vi "DPO_7K_Read Multiple Waveforms.vi"(8 "error in (no error)":errorcluster, 10 "Channels":u16[](array[ring])=[0] items=["Channel 1", "Channel 2", "Channel 3", "Channel 4", "Math 1", "Math 2", "Math 3", "Math 4", "Reference 1", "Reference 2", "Reference 3", "Reference 4"], 11 "VISA resource name":refnum<visa-resource-name>) -> (0 "error out":errorcluster, 1 "ChannelsArray":u16[](array[ring]) caption="Channels" items=["Channel 1", "Channel 2", "Channel 3", "Channel 4", "Math 1", "Math 2", "Math 3", "Math 4", "Reference 1", "Reference 2", "Reference 3", "Reference 4"], 2 "Waveform Data":waveform(dbl)[](graph), 3 "VISA resource name out":refnum<visa-resource-name>)   [LabVIEW 2020]
doc: "Initiates an acquisition on all channels that you enabled with the Configure Channel VI. This VI waits for the acquisition to complete and returns the waveform for the <B>Channel</B> you specify. If the oscilloscope does not complete the acquisition within the <B>Maximum Time</B> period, this VI returns a timeout error. A timeout error often occurs because the acquisition is not triggered. For example, if the trigger level is out of range of the waveform, the acquisition is not triggered.\n\nRun the Fetch Waveform VI to obtain the waveforms for each of the remaining enabled <B>Channels</B> without initiating another acquisition.\n\n<B>Note:</B> If the instrument does not support autocompensation for probe attenuation, you might need to adjust the scaling of the <B>Waveform Data</B> accordingly. You can adjust the scaling using the Configure Channel VI or manually multiplying the <B>Waveform Data</B> by the probe attenuation."
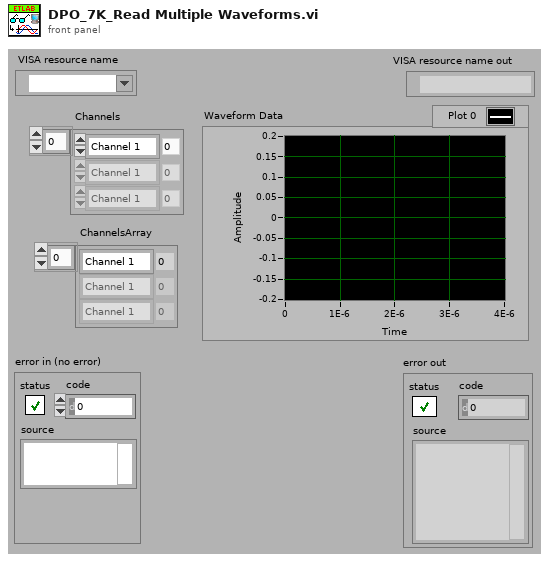
[diagram p1: front panel]
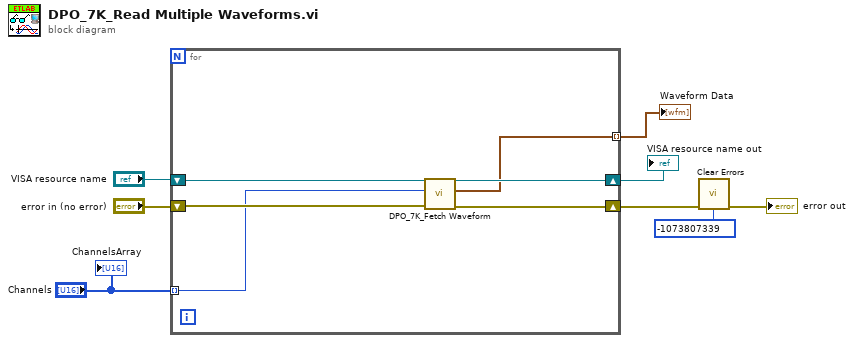
[diagram p0: block diagram]
diagram:
  n1 = for {
    shift-right: [w13] -> w3
    shift-left: "error in (no error)" -> [w11]
    shift-right: [w14] -> w8
    shift-left: "VISA resource name" -> [w12]
    tunnel: [w10] -> w7 mode=indexing
    tunnel: "Channels" -> [w9] mode=indexing
    n2 = call "DPO_7K_Fetch Waveform.vi"("error in (no error)"=w11, "Channel (0:Channel1)"=w9, "VISA resource name"=w12) -> ("error out"=w13:errorcluster, "Waveform Data"=w10:waveform(dbl), "VISA resource name out"=w14:refnum<visa-resource-name>)  [unwired: 6 in]
  }
  "VISA resource name out" <- w8
  "Waveform Data" <- w7
  n3 = call <vilib>:"Clear Errors.vi"("error in (no error)"=w3, "specific error code to clear (0: all)"=-1073807339) -> ("error out"=→"error out":errorcluster)  [unwired: 4 in, 1 out]
  "ChannelsArray" <- "Channels"
